vi "Test A.vi"(7 "Socket":i32, 8 "error in (no error)":errorcluster) -> (0 "error out":errorcluster)   [LabVIEW 2019, in "Multisocket Example(Station2).lvlib"]
uses:
  Multisocket Example(Station2).lvlib
  d31799f9-9e59-4a03-9ea0-60b3ce935fd9.vi
  00355e06-9aa9-4587-985a-8f165454d30f.vi
  LVUT Global 1.vi
  <vilib>/Utility/Data Type/Get Type Information.vi
  Almost Equal.vi
  Unit Test Engine Tools.lvlib
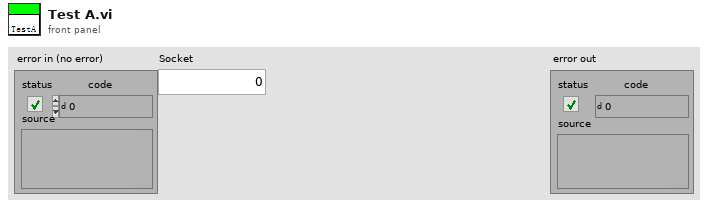
[diagram p1: front panel]
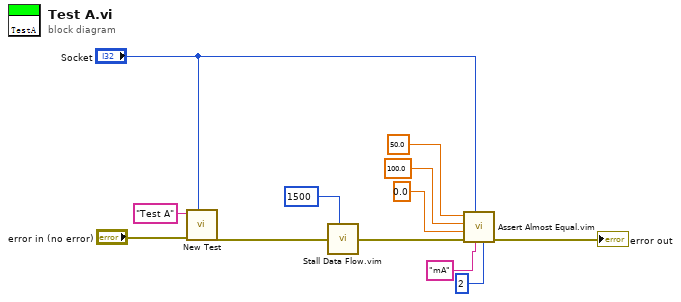
[diagram p0: block diagram]
diagram:
  n1 = call "New Test.vi"("Socket"="Socket", "error in (no error)"="error in (no error)", "Test"="Test A") -> ("error out"=w10:errorcluster)  [unwired: 8 in]
  n2 = call "Stall Data Flow.vim"("value in"=w10, "milliseconds to wait"=u32 1500) -> ("value out"=w8:errorcluster)  [unwired: 1 out]
  n3 = call "Assert Almost Equal.vim"("precision (2)"=i16 2 ("precision (6)"), "Unit"="mA", "Socket"="Socket", "error in (no error)"=w8, "a"=0.0 ("Low limit"), "b"=100.0 ("High limit"), "x"=50.0 ("X")) -> ("error out"=→"error out":errorcluster)  [unwired: 4 in]
